vi "Player Info.vi"(11 "SquareA in":refnum<class "Ant Mound.lvclass">) -> (0 "Defeat Speech":string, 1 "Victory Speech":string, 2 "Name":string, 3 "SquareA out":refnum<class "Ant Mound.lvclass">)   [LabVIEW 2017, in "Ant Mound.lvclass"]
uses:
  Ant Mound.lvclass
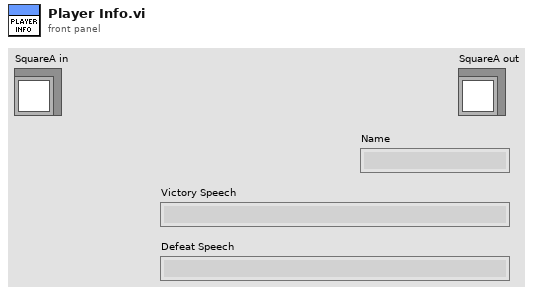
[diagram p1: front panel]
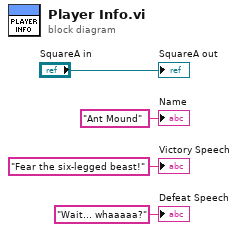
[diagram p0: block diagram]
diagram:
  "SquareA out" <- "SquareA in"
  "Name" <- "Ant Mound" ("Name")
  "Victory Speech" <- "Fear the six-legged beast!" ("Victory Speech")
  "Defeat Speech" <- "Wait... whaaaaa?" ("Defeat Speech")
